vi "写入数据库.vi"(0 "数据显示":refnum<vi>, 2 "错误输入（无错误）":errorcluster) -> (1 "错误输出":errorcluster)   [LabVIEW 2015]
panel:
  in  "数据显示":string[][](table)
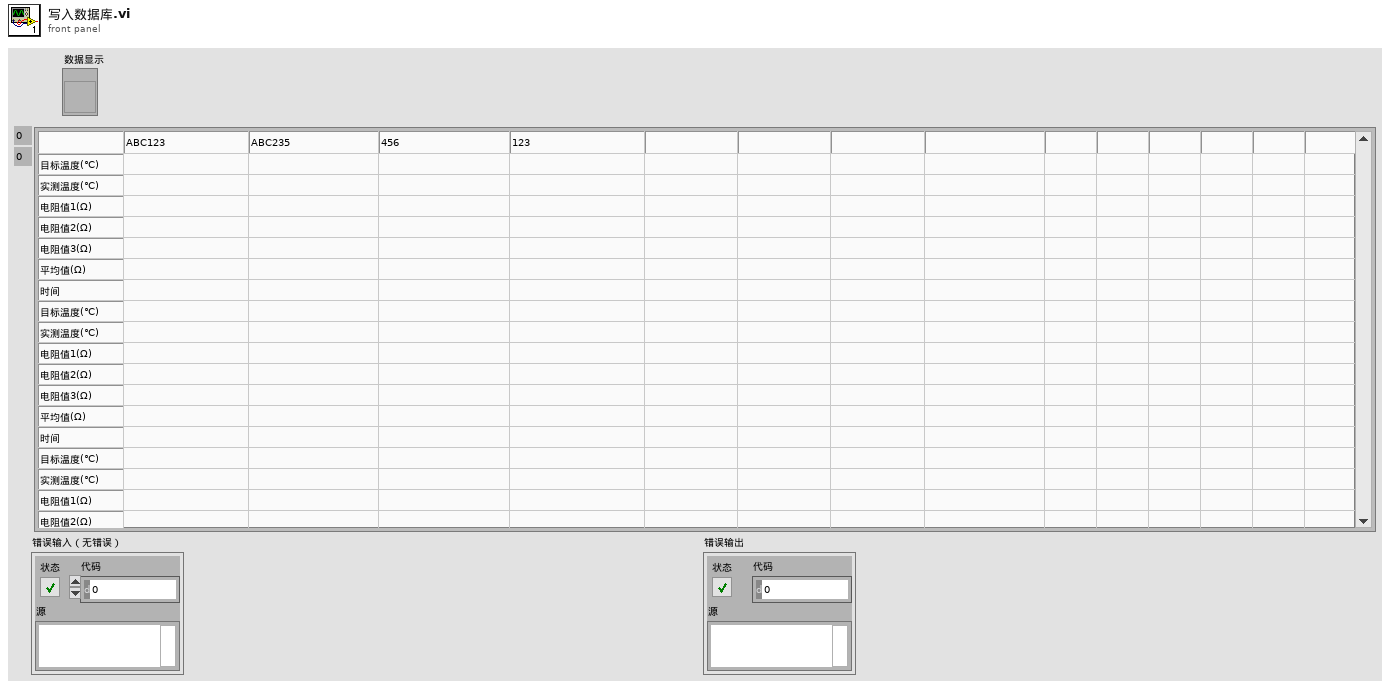
[diagram p1: front panel]
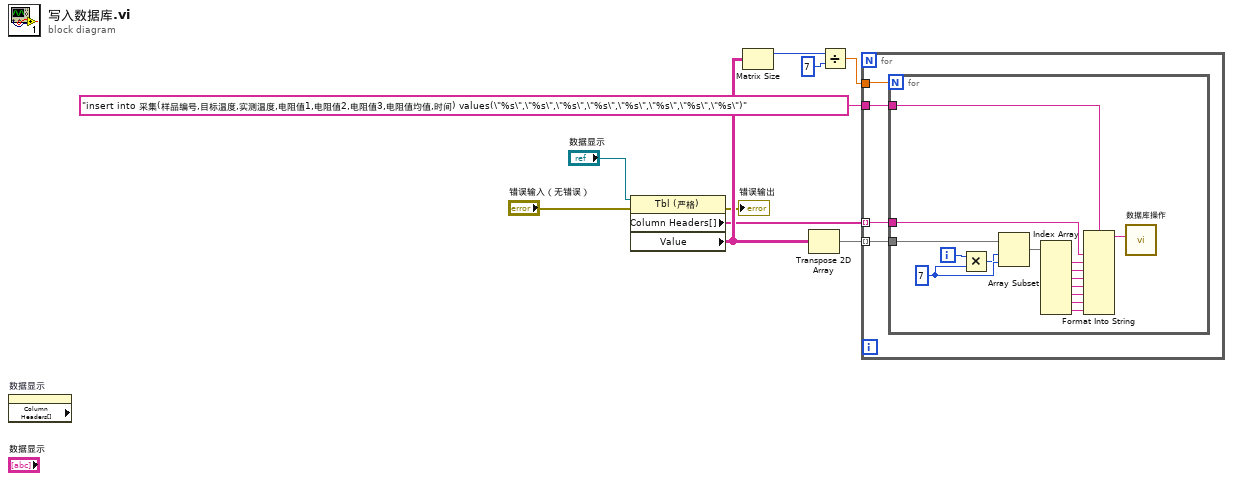
[diagram p0: block diagram]
diagram:
  n1 = property on="数据显示" class="Tbl (严格)" props=["Column Headers[]"]() -> ()  [unwired: 2 in, 3 out]
  n2 = property class="Tbl (严格)"(reference="数据显示", error in="错误输入（无错误）") -> (error out=→"错误输出":errorcluster, "Column Headers[]"=w3:string[], "Value"=w4:string[][])  [unwired: 1 out]
  n3 = Matrix Size(0:w4) -> (1:w9:i32)  [unwired: 1 out]
  n4 = Transpose 2D Array(2D array=w4) -> (transposed array=w10:string[][])
  n5 = Divide(x=w9, y=7 ("长度")) -> (x/y=w7:dbl)
  n6 = for {
    tunnel: w10 -> [w14] mode=indexing
    tunnel: w3 -> [w12] mode=indexing
    tunnel: w7 -> [w13]
    tunnel: "insert into 采集(样品编号,目标温度,实测温度,电阻值1,电阻值2,电阻值3,电阻值均值,时间) values(\"%s\",\"%s\",\"%s\",\"%s\",\"%s\",\"%s\",\"%s\",\"%s\")" ("SQL") -> [w11]
    n7 = for {
      N: w13 -> [_]
      tunnel: w14 -> [w29]
      tunnel: w12 -> [w25]
      tunnel: w11 -> [w16]
      i -> [w28]
      w27 = 7 ("长度")
      n8 = Multiply(x=w28, y=w27) -> (x*y=w26:i32)
      n9 = Array Subset(array=w29, index=w26, length=w27) -> (w24:string[])
      n10 = Index Array(array=w24) -> (element #1=w23:string, element #2=w22:string, element #3=w21:string, element #4=w20:string, element #5=w19:string, element #6=w18:string, element #7=w15:string)  [unwired: 7 in]
      n11 = Format Into String(format string=w16, w25, w23, w22, w21, w20, w19, w18, w15) -> (resulting string=w17:string)  [unwired: 2 in, 1 out]
      n12 = call "数据库操作.vi"("SQL query"=w17) -> ()  [unwired: 9 in, 2 out]
    }
  }
